vi "BELKIN Fill Source FIFO.vi"(7 "Write Timeout (ms)":i32=5000, 8 "error in (no error)":errorcluster, 9 "FPGA VI Reference In":T1, 10 "Maximum Pixels per Write":i32=-1, 11 "Image":T2) -> (0 "error out":errorcluster, 1 "FPGA VI Reference Out":T1, 3 "Image Out":T2)   [LabVIEW 2015]
doc: "Transfers an image from the host processor to the target FPGA via a DMA FIFO."
uses:
  <vilib>/vision/Image Controls.llb/IMAQ Image.ctl
  Controls/FPGA IP Chain V1 Ref.ctl
  <vilib>/rvi/errors/niLvFpgaAdjustHostInterfaceError.vi
  <vilib>/rvi/interface/nirviMethod/nirviMethod.xnode
  FPGA Bitfiles/BELKINEAGLE_FPGATarget_FPGAIPChainV1_CFyF0ro37YQ.lvbitx
  FPGA IP Chain V1.vi
  nivissvc.dll
  <vilib>/rvi/errors/niLvFpgaMergeErrorWithErrorCode.vi
  <vilib>/FPGAPlugInAG/cRIO-9030/niLvFpga_WriteFifo_cRIO-9030.vi
  <vilib>/FPGAPlugInAG/cRIO-9030/niLvFpga_AcquireWriteRegionFifo_cRIO-9030.vi
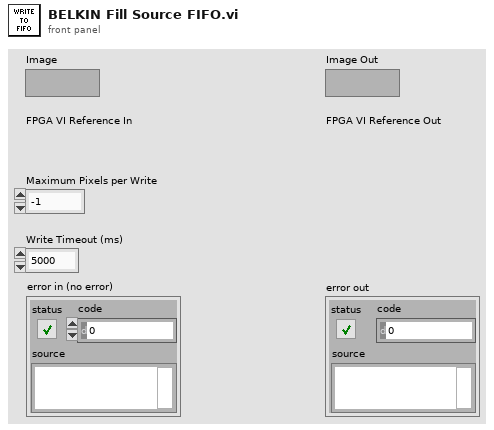
[diagram p1: front panel]
types:
  T1 = typedef "FPGA IP Chain V1 Ref.ctl" = refnum<k20>
  T2 = typedef "IMAQ Image.ctl" = refnum<image>
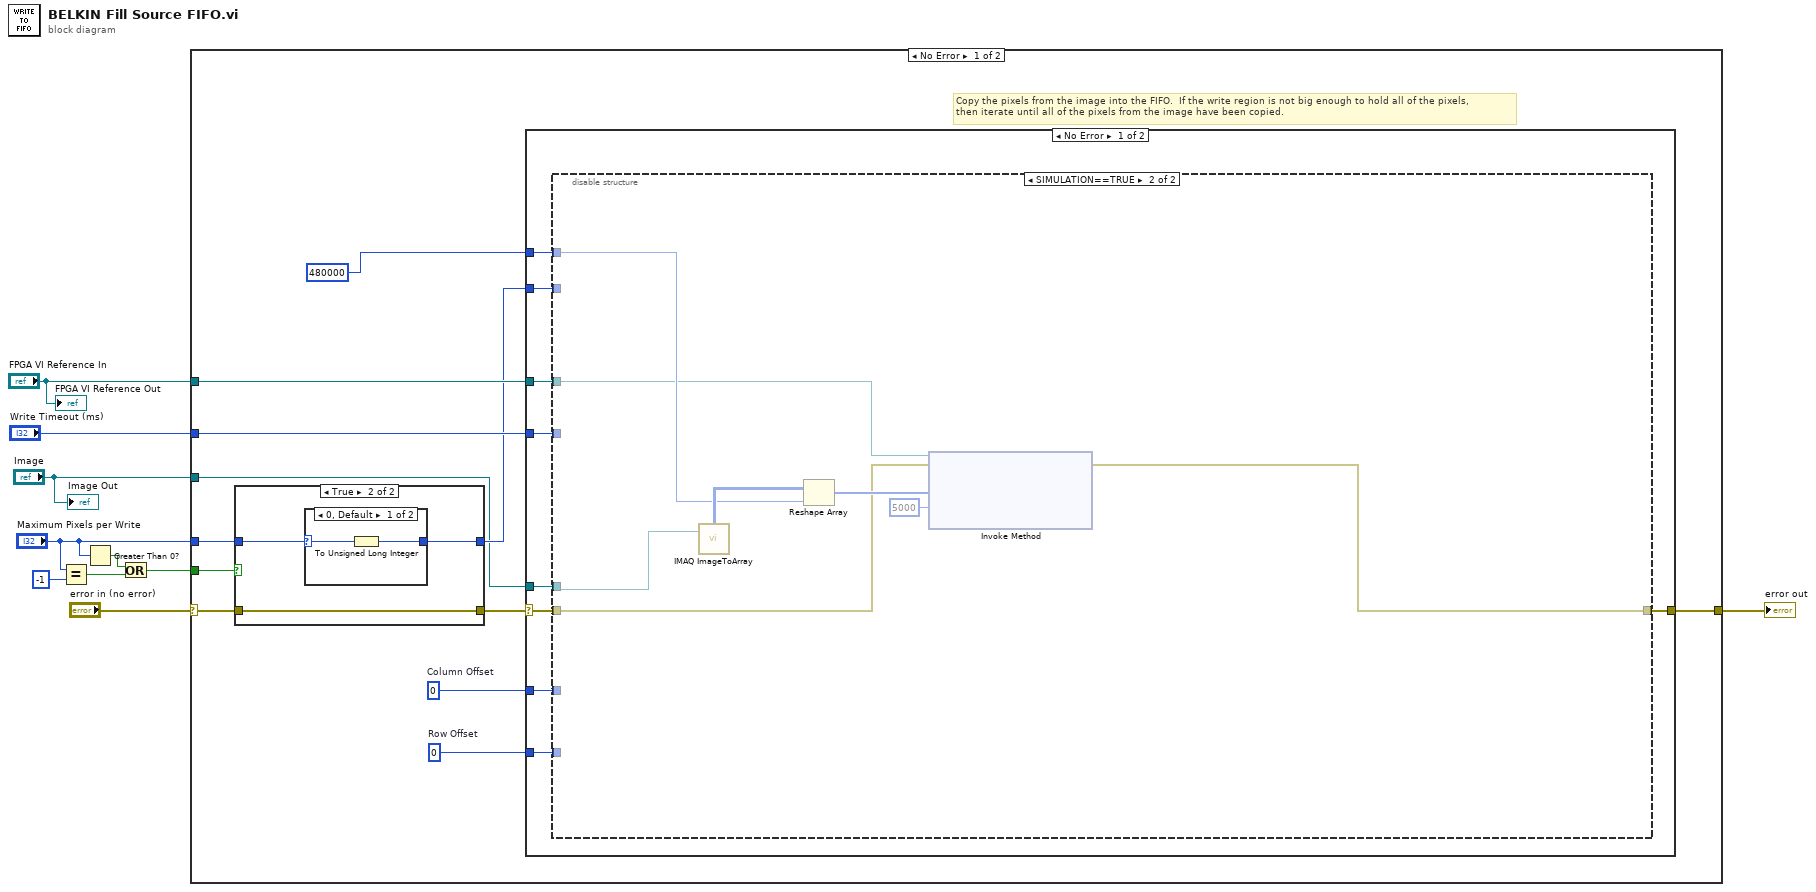
[diagram p0: block diagram]
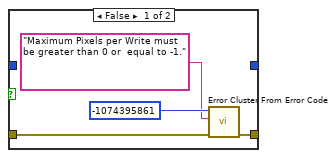
[diagram p2: hidden frame]
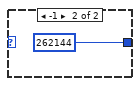
[diagram p3: hidden frame]
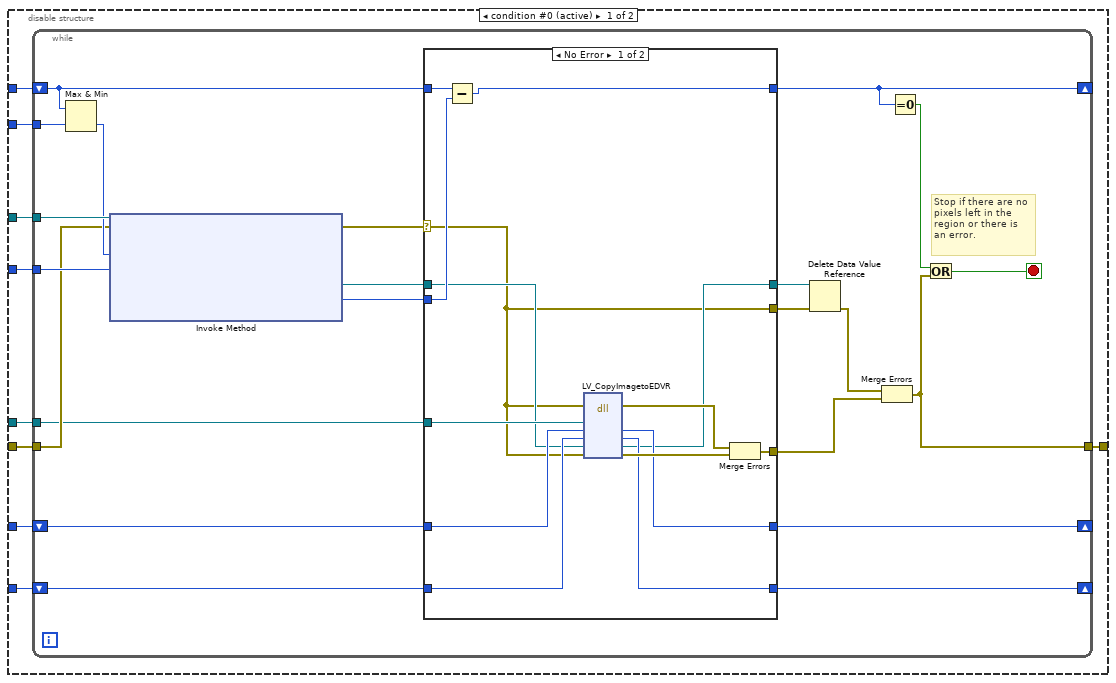
[diagram p4: hidden frame]
diagram:
  n1 = Equal?(x="Maximum Pixels per Write", y=-1) -> (x = y?=w6:bool)
  n2 = Greater Than 0?(x="Maximum Pixels per Write") -> (x > 0?=w7:bool)
  n3 = Or(x=w7, y=w6) -> (x .or. y?=w5:bool)
  n4 = case shown="No Error" "error in (no error)" {
    selector: "error in (no error)" -> [w12 w101]
    tunnel: "FPGA VI Reference In" -> [w22 _]
    tunnel: "Write Timeout (ms)" -> [w21 _]
    tunnel: w5 -> [w18 _]
    tunnel: "Maximum Pixels per Write" -> [w15 _]
    tunnel: "Image" -> [w14 _]
    tunnel: [w13 w101] -> w2
    frame No Error {
      w19 = u32 0  # Row Offset
      w20 = u32 0  # Column Offset
      # "Copy the pixels from the image into the FIFO.  If the write region is not big enough to hold all of the pixels,\nthen iterate until all of the pixels from the image have been copied."
      n5 = case shown="True" w18 {
        tunnel: w12 -> [w24 w29]
        tunnel: [w23 w29] -> w17
        tunnel: w15 -> [_ w28]
        tunnel: [_ w27] -> w16
        frame False {
          n6 = call <vilib>:"Error Cluster From Error Code.vi"("error in (no error)"=w24, "error message (\"\")"="Maximum Pixels per Write must be greater than 0 or  equal to -1." ("error message (\"\")"), "error code (0)"=-1074395861) -> ("error out"=w23:errorcluster)  [unwired: 6 in]
        }
        frame True {
          n7 = case shown="0, Default" w28 {
            selector: w28 -> [w31 _]
            tunnel: [w30 u32 262144 ("Maximum Pixels per Write")] -> w27
            frame 0, Default {
              n8 = To Unsigned Long Integer(number=w31) -> (unsigned 32bit integer=w30:u32)
            }
            frame -1 {
            }
          }
        }
      }
      n9 = case shown="No Error" w17 {
        selector: w17 -> [w35 w100]
        tunnel: 480000 ("x*y") -> [w41 _]
        tunnel: w20 -> [w37 _]
        tunnel: w19 -> [w36 _]
        tunnel: w22 -> [w39 _]
        tunnel: [w33 w100] -> w13
        tunnel: w16 -> [w40 _]
        tunnel: w21 -> [w38 _]
        tunnel: w14 -> [w34 _]
        frame No Error {
          n10 = disable-structure shown="SIMULATION==TRUE" {
            disable-tunnel: w41 -> [w50 w97]
            disable-tunnel: w40 -> [w49 _]
            disable-tunnel: w39 -> [w48 w96]
            disable-tunnel: w38 -> [w47 _]
            disable-tunnel: w37 -> [w46 _]
            disable-tunnel: w36 -> [w45 _]
            disable-tunnel: w35 -> [w44 w92]
            disable-tunnel: w34 -> [w43 w99]
            disable-tunnel: [w42 w93] -> w33
            frame condition #0 (active) {
              n11 = while {
                shift-right: [w60] -> _
                shift-left: w50 -> [w55]
                shift-right: [w67] -> _
                shift-left: w46 -> [w69]
                shift-right: [w70] -> _
                shift-left: w45 -> [w68]
                tunnel: w48 -> [w66]
                tunnel: [w58] -> w42
                tunnel: w49 -> [w54]
                tunnel: w47 -> [w53]
                tunnel: w44 -> [w52]
                tunnel: w43 -> [w51]
                stop <- w59 stop-if-true
                # "Stop if there are no\npixels left in the \nregion or there is\nan error."
                n12 = Max & Min(x=w55, y=w54) -> (min(x,y)=w56:u32)  [unwired: 1 out]
                n13 = xnode "Invoke Method"("FPGA VI Reference In"=w66, "error in"=w52, "Number of Elements"=w56, "Timeout (ms)"=w53) -> ("error out"=w65:errorcluster, "Write Region Reference"=w72:refnum<data-value>, "Elements In Region"=w71:u32)  [unwired: 2 out]
                n14 = case shown="No Error" w65 {
                  selector: w65 -> [w73 w88]
                  tunnel: w55 -> [w86 w91]
                  tunnel: [w85 w91] -> w60
                  tunnel: w72 -> [w79 w87]
                  tunnel: w71 -> [w84 _]
                  tunnel: [w75 w89] -> w70
                  tunnel: w69 -> [w82 w90]
                  tunnel: w68 -> [w81 w89]
                  tunnel: [w76 w90] -> w67
                  tunnel: [w74 w87] -> w64
                  tunnel: [w73 w88] -> w63
                  tunnel: [w77 _] -> w61
                  tunnel: w51 -> [w83 _]
                  frame No Error {
                    n15 = Subtract(x=w86, y=w84) -> (x-y=w85:u32)
                    n16 = dll-call lib="nivissvc.*" fn="LV_CopyImagetoEDVR" label="LV_CopyImageToEDVR"(error in=w73, "image"=w83, "xImageOffset"=w82, "yImageOffset"=w81, "EDVR"=w79, "error"=w73) -> (error out=w80:errorcluster, "xImageOffset"=w76:u32, "yImageOffset"=w75:u32, "EDVR"=w74:refnum<data-value>, "error"=w78:errorcluster)  [unwired: 4 in, 1 out]
                    n17 = Merge Errors(w80, w78) -> (w77:errorcluster)
                  }
                  frame Error {
                  }
                }
                n18 = Delete Data Value Reference(data value reference=w64, error in=w63) -> (error out=w62:errorcluster)  [unwired: 1 out]
                n19 = Merge Errors(w62, w61) -> (w58:errorcluster)
                n20 = Equal To 0?(x=w60) -> (x = 0?=w57:bool)
                n21 = Or(x=w57, y=w58) -> (x .or. y?=w59:bool)
              }
            }
            frame condition #1 {
              n22 = call "IMAQ ImageToArray"("Image"=w99) -> ("Image Pixels (U8)"=w98:u8[][])  [unwired: 3 in, 4 out]
              n23 = Reshape Array(w98, w97) -> (w95:u8[])
              n24 = xnode "Invoke Method"("FPGA VI Reference In"=w96, "error in"=w92, "Data"=w95, "Timeout (ms)"=5000) -> ("error out"=w93:errorcluster)  [unwired: 2 out]
            }
          }
        }
        frame Error {
        }
      }
    }
    frame Error {
    }
  }
  "error out" <- w2
  "Image Out" <- "Image"
  "FPGA VI Reference Out" <- "FPGA VI Reference In"
